vi "FXP NILIA_VCO.vi"(9 "nominal freq [U16.0]":fxp<+,16,0>, 10 "Kv [U16.0]":fxp<+,16,0>, 11 "v [I32.17]":fxp<+/-,32,17>) -> (0 "f":fxp<+/-,32,0> format="%.32g", 1 "z [I32.1]":fxp<+/-,32,1>, 2 "sin(z) [I16.2]":fxp<+/-,16,2> format="%.15g", 3 "cos(z) [I16.2]":fxp<+/-,16,2> format="%.15g")   [LabVIEW 2009]
uses:
  <vilib>/rvi/FXPMathLib/FxpMul/XNode/nifxpmath_Multiplier.xnode
  <vilib>/rvi/FXPMathLib/FxpMul/subVIs/nifxpmath_Mul_SimConfig.ctl
  <vilib>/fxp/LVFixedPointQuantizationPolicyTypeDef.ctl
  <vilib>/fxp/LVFixedPointOverflowPolicyTypeDef.ctl
  <vilib>/rvi/FXPMathLib/FxpMul/simVIs/DllFxpMulTemp_sub.vi
  <vilib>/rvi/FXPMathLib/FxpAdd/XNode/nifxpmath_Add.xnode
  <vilib>/rvi/FXPMathLib/FxpAdd/subVIs/nifxpmath_Add_SimConfig.ctl
  <vilib>/rvi/FXPMathLib/FxpAdd/simVIs/DllFxpAddTemp_sub.vi
  <vilib>/rvi/FXPMathLib/basic elements/FxpIntAccumulator/XNode/nifxpmath_IntAccumulator.xnode
  <vilib>/rvi/FXPMathLib/basic elements/FxpIntAccumulator/subVIs/nifxpmath_IntAccumulator_SimConfig.ctl
  <vilib>/rvi/FXPMathLib/basic elements/FxpIntAccumulator/simVIs/DllFxpIntAccumulator_sub.vi
  <vilib>/rvi/FXPMathLib/FxpSinAndCos/XNode/nifxpmath_SinAndCos.xnode
  <vilib>/rvi/FXPMathLib/FxpSinAndCos/subVIs/nifxpmath_SinAndCos_SimConfig.ctl
  <vilib>/rvi/FXPMathLib/FxpSinAndCos/simVIs/DllFxpSinAndCosTemp_sub.vi
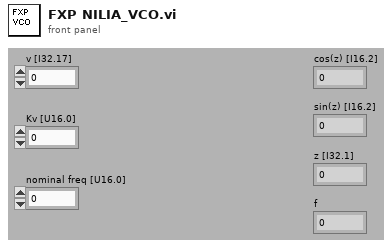
[diagram p1: front panel]
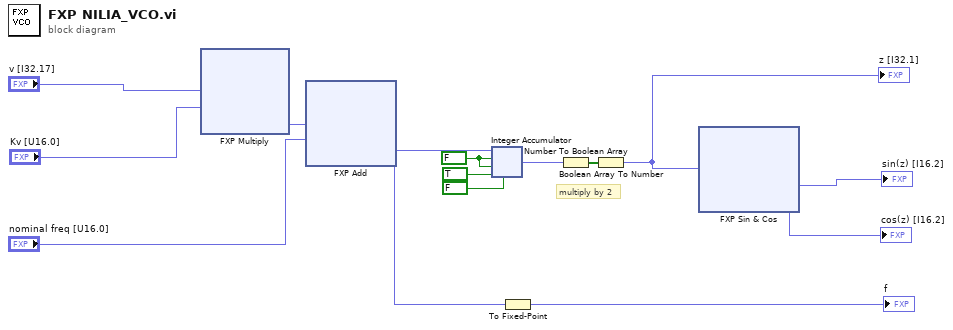
[diagram p0: block diagram]
diagram:
  w8 = FALSE ("is sub")
  # "multiply by 2"
  n1 = xnode "FXP Multiply"("x"="v [I32.17]", "y"="Kv [U16.0]") -> ("x*y"=w5:fxp<+/-,32,0>)
  n2 = xnode "FXP Add"("x"=w5, "y"="nominal freq [U16.0]") -> ("x+y"=w3:fxp<+/-,32,0>)
  n3 = xnode "Integer Accumulator"("x"=w3, "load"=w8, "is sub?"=w8, "enable"=TRUE, "carry-in/inverted borrow-in"=FALSE ("cin/nbin")) -> ("s"=w2:fxp<+/-,32,0>)  [unwired: 1 out]
  n4 = To Fixed-Point(number=w3) -> (fixed-point=→"f":fxp<+/-,32,0>)  [unwired: 1 out]
  n5 = Number To Boolean Array(number=w2) -> (Boolean array=w4:bool[])
  n6 = Boolean Array To Number(Boolean array=w4) -> (number=w10:fxp<+/-,32,1>)
  "z [I32.1]" <- w10
  n7 = xnode "FXP Sin & Cos"("x (pi)"=w10) -> ("sin(x)"=→"sin(z) [I16.2]":fxp<+/-,16,2>, "cos(x)"=→"cos(z) [I16.2]":fxp<+/-,16,2>)
